vi "process.vi"(8 "error in (no error)":errorcluster, 11 "Subscription in":refnum<class "Subscription.lvclass">) -> ()   [LabVIEW 2013, in "MQTT Server.lvlib" / "Subscription.lvclass"]
uses:
  Subscription.lvclass
  Subscription.lvclass/Subscription.ctl
  TopicFilter/TopicFilter.lvclass/TopicFilter.ctl
  TopicFilter/TopicFilter.lvclass
  Control Packets/PUBLISH/PUBLISH.lvclass
panel:
  out "Topic Filter":string
  out "Numeric":i32
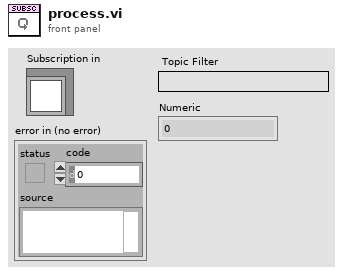
[diagram p1: front panel]
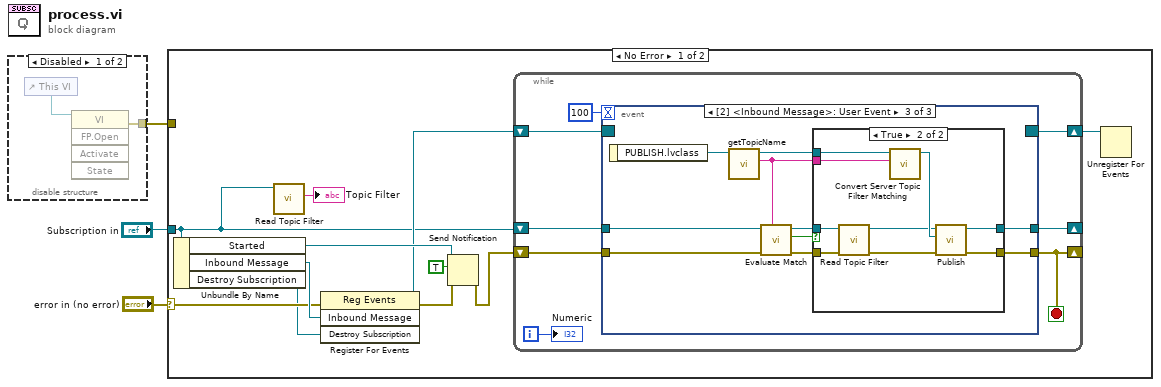
[diagram p0: block diagram]
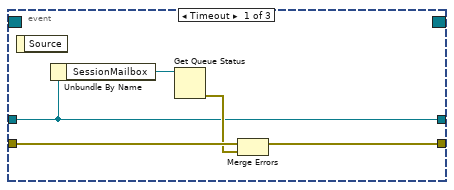
[diagram p3: hidden frame]
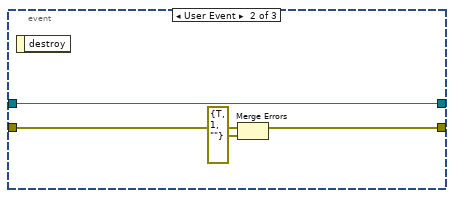
[diagram p4: hidden frame]
diagram:
  n1 = disable-structure shown="Disabled" {
    disable-tunnel: [w4 _] -> w1
    frame Disabled {
      n2 = control-ref of="This VI"() -> (w5:refnum<vi>)
      n3 = invoke class="VI" method="FP.Open"(reference=w5) -> (error out=w4:errorcluster)  [unwired: 4 in, 4 out]
    }
    frame Enabled {
    }
  }
  n4 = case shown="No Error" "error in (no error)" {
    selector: "error in (no error)" -> [w12 _]
    tunnel: "Subscription in" -> [w8 _]
    tunnel: w1 -> [_ _]
    frame No Error {
      n5 = Unbundle By Name(w8) -> ("Started"=w14:refnum<notifier>, "Inbound Message"=w13:refnum<user-event>, "Destroy Subscription"=w6:refnum<user-event>)
      n6 = call "Read Topic Filter.vi"("Subscription in"=w8) -> ("Topic Filter"=→"Topic Filter":string)  [unwired: 7 in, 3 out]
      n7 = register-events(error in=w12, w13, w6) -> (reference out=w10:refnum<event-registration>, error out=w11:errorcluster)  [unwired: 1 in]
      n8 = Send Notification(notification=TRUE, notifier=w14, error in (no error)=w11) -> (error out=w15:errorcluster)  [unwired: 1 out]
      n9 = while {
        shift-right: [w19] -> _
        shift-left: w15 -> [w20]
        shift-right: [w22] -> w9
        shift-left: w10 -> [w23]
        shift-right: [w17] -> _
        shift-left: w8 -> [w21]
        i -> [w18]
        stop <- w19 stop-if-true
        n10 = event shown="[2] <Inbound Message>: User Event" {
          selector: w23 -> [_ _ _]
          dyn-events: [_ _ _] -> w22
          timeout: 100 -> [_ _ _]
          tunnel: w21 -> [w25 w31 w41]
          tunnel: w20 -> [w28 w33 w42]
          tunnel: [w26 w32 w43] -> w19
          tunnel: [w25 w31 w35] -> w17
          event Timeout {
            n11 = event-data() -> ()  [unwired: 1 in, 1 out]
            n12 = Unbundle By Name(w25) -> ("SessionMailbox"=w29:refnum<queue>)
            n13 = Get Queue Status(queue=w29) -> (error out=w27:errorcluster)  [unwired: 2 in, 7 out]
            n14 = Merge Errors(w28, w27) -> (w26:errorcluster)
          }
          event User Event {
            n15 = event-data() -> ()  [unwired: 1 in, 1 out]
            n16 = Merge Errors(w33, errorcluster {"status"=TRUE, "code"=1, "source"=""} ("error in")) -> (w32:errorcluster)
          }
          event User Event {
            n17 = event-data() -> ("PUBLISH.lvclass"=w40:refnum<class "PUBLISH.lvclass">)  [unwired: 1 in]
            n18 = call "getTopicName.vi"("PUBLISH in"=w40) -> ("Topic"=w34:string, "PUBLISH out"=w39:refnum<class "PUBLISH.lvclass">)  [unwired: 8 in, 1 out]
            n19 = call "Evaluate Match.vi"("Topic"=w34, "error in (no error)"=w42, "Subscription in"=w41) -> ("error out"=w36:errorcluster, "Matched"=w38:bool, "Subscription out"=w37:refnum<class "Subscription.lvclass">)  [unwired: 5 in, 1 out]
            n20 = case shown="True" w38 {
              tunnel: [w45 w54] -> w43
              tunnel: w36 -> [w45 w48]
              tunnel: w37 -> [w44 w50]
              tunnel: w39 -> [_ w52]
              tunnel: [w44 w53] -> w35
              tunnel: w34 -> [_ w46]
              frame False {
              }
              frame True {
                n21 = call "Read Topic Filter.vi"("error in (no error)"=w48, "Subscription in"=w50) -> ("error out"=w47:errorcluster, "Subscription out"=w49:refnum<class "Subscription.lvclass">)  [unwired: 6 in, 2 out]
                n22 = call "Convert Server Topic Filter Matching.vi"("Matching Topic Filter"=w46, "PUBLISH"=w52) -> ("Server PUBLISH"=w51:refnum<class "PUBLISH.lvclass">)  [unwired: 8 in, 1 out]
                n23 = call "Publish.vi"("error in (no error)"=w47, "PUBLISH"=w51, "Subscription in"=w49) -> ("error out"=w54:errorcluster, "Subscription out"=w53:refnum<class "Subscription.lvclass">)  [unwired: 7 in]
              }
            }
          }
        }
        "Numeric" <- w18
      }
      n24 = Unregister For Events(event registration refnum=w9) -> ()  [unwired: 1 in, 1 out]
    }
    frame Error {
    }
  }
